vi "Generate Header Vectors.vi"(0 "RFFE Reg0Write Command in":refnum<class "RFFE Reg0Write Command.lvclass">, 11 "error in (no error)":errorcluster) -> (4 "RFFE Reg0Write Command out":refnum<class "RFFE Reg0Write Command.lvclass">, 6 "Header Vectors":string[](array[string]), 15 "error out":errorcluster)   [LabVIEW 2018, in "MIPI RFFE API.lvlib" / "RFFE Reg0Write Command.lvclass"]
uses:
  RFFE Reg0Write Command.lvclass
  RFFE Reg0Write Command.lvclass/RFFE Reg0Write Command.ctl
  Command/RFFE Command.lvclass
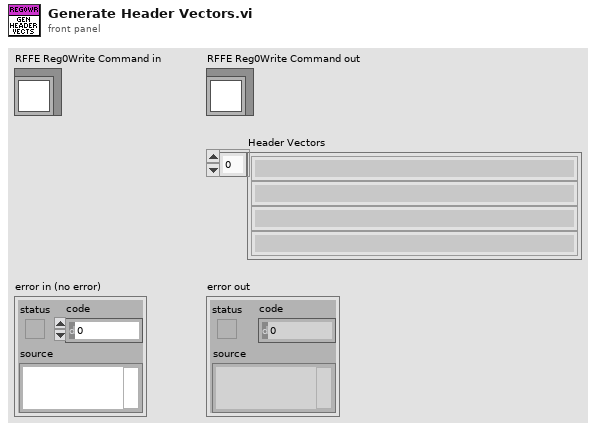
[diagram p1: front panel]
types:
  T1 = typedef "MIPI RFFE API.lvlib/Register Data.ctl" = u8
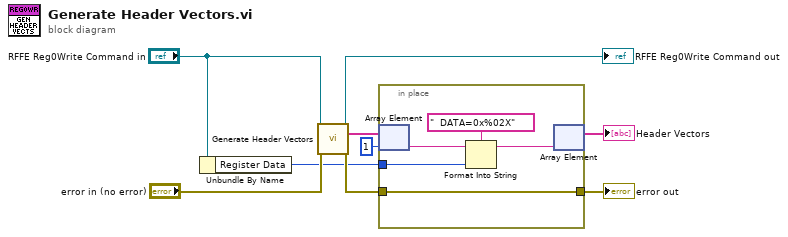
[diagram p0: block diagram]
diagram:
  n1 = Unbundle By Name("RFFE Reg0Write Command in") -> ("Register Data"=w1:T1)
  n2 = call-parent "Generate Header Vectors.vi"("RFFE Command in"="RFFE Reg0Write Command in", "error in (no error)"="error in (no error)") -> ("RFFE Command out"=→"RFFE Reg0Write Command out":refnum<class "RFFE Reg0Write Command.lvclass">, "Header Vectors"=w9:string[], "error out"=w3:errorcluster)  [unwired: 11 in]
  n3 = in-place {
    in-place-border: w3 -> [w13]
    in-place-border: [w13] -> w2
    in-place-border: w1 -> [w10]
    n4 = in-place-array #1(w9, 1) -> (w12:string)
    n5 = Format Into String(format string="  DATA=0x%02X", initial string=w12, w10) -> (resulting string=w11:string)  [unwired: 1 in, 1 out]
    n6 = in-place-array #1(w11) -> (→"Header Vectors":string[])  [unwired: 1 out]
  }
  "error out" <- w2
